vi "hydraharp_initialize_correlation.vi"(8 "error in (no error)":errorcluster, 11 "hydraharp in":refnum<class "hydraharp.lvclass">) -> (0 "error out":errorcluster, 3 "hydraharp out":refnum<class "hydraharp.lvclass">)   [LabVIEW 2015, in "hydraharp.lvclass"]
uses:
  hydraharp.lvclass
  hydraharp.lvclass/hydraharp.ctl
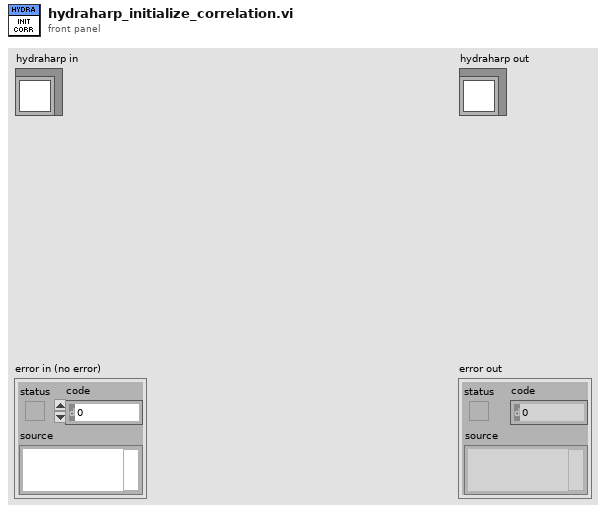
[diagram p1: front panel]
types:
  T1 = cluster{"log_bin_edges":dbl[], "ch1_photons":dbl[], "ch2_photons":dbl[], "elements_in_record_buffers":i32[], "number_of_new_photons":i32[]}
  T2 = typedef "hydraharp_correlation_lag_settings.ctl" = cluster{"time_start":T3, "time_end":T3, "coarseness":i64}
  T3 = typedef "hydraharp_time_decades.ctl" = i64
  T4 = typedef "hydraharp_action_on_records.ctl" = enum16{"stream_to_file", "correlate", "stream to file and correlate"}
  T5 = typedef "hpanel_acq_modes.ctl" = u16
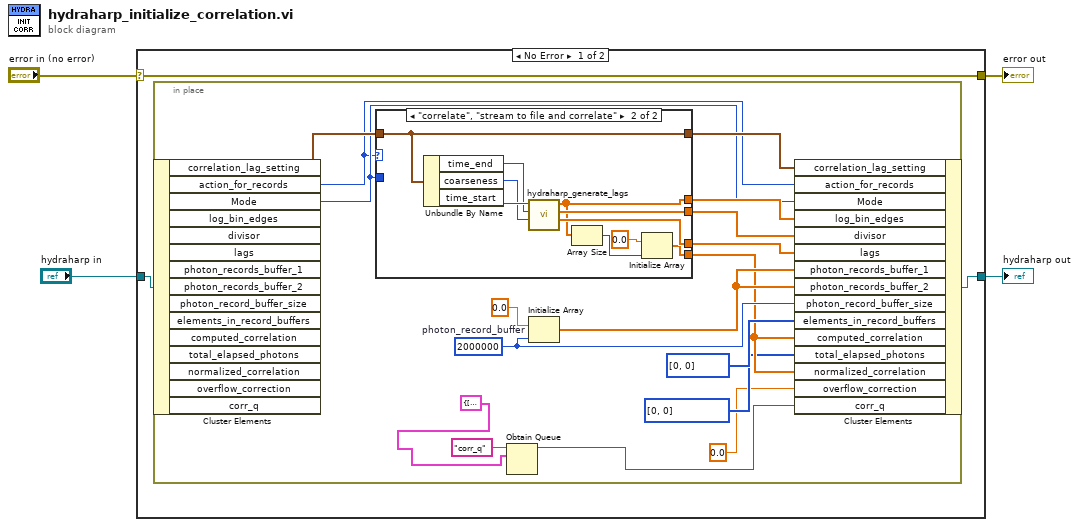
[diagram p0: block diagram]
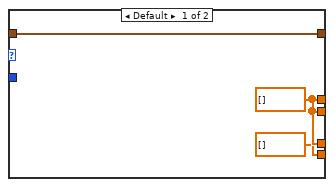
[diagram p2: hidden frame]
diagram:
  n1 = case shown="No Error" "error in (no error)" {
    selector: "error in (no error)" -> [w7 w39]
    tunnel: [w7 w39] -> w3
    tunnel: [w5 w38] -> w1
    tunnel: "hydraharp in" -> [w6 w38]
    frame No Error {
      n2 = in-place {
        w15 = 2000000 ("dimension size")
        n3 = in-place-cluster #1(w6) -> ("correlation_lag_setting"=w24:T2, "action_for_records"=w18:T4, "Mode"=w19:T5)  [unwired: 12 out]
        n4 = case shown="\"correlate\", \"stream to file and correlate\"" w18 {
          tunnel: w19 -> [_ _]
          tunnel: w24 -> [w27 w34]
          tunnel: [w27 w34] -> w23
          tunnel: [w26 w33] -> w22
          tunnel: [w26 w30] -> w21
          tunnel: [w26 w32] -> w20
          tunnel: [dbl[] [] w28] -> w13
          frame Default {
            w26 = dbl[] [] ("lags")
          }
          frame "correlate", "stream to file and correlate" {
            n5 = Unbundle By Name(w34) -> ("time_end"=w35:T3, "coarseness"=w36:i64, "time_start"=w37:T3)
            n6 = call "hydraharp_generate_lags.vi"("coarseness"=w36, "time_end"=w35, "time_start"=w37) -> ("lags"=w32:dbl[], "divisor"=w33:dbl[], "log_bin_edges"=w30:dbl[])  [unwired: 6 in]
            n7 = Array Size(array=w30) -> (size(s)=w29:i32)
            n8 = Initialize Array(0.0 ("element"), w29) -> (w28:dbl[])
          }
        }
        n9 = Obtain Queue(name (unnamed)="corr_q", element data type=T1 {"log_bin_edges"=[], "ch1_photons"=[], "ch2_photons"=[], "elements_in_record_buffers"=[], "number_of_new_photons"=[]} ("output cluster")) -> (queue out=w8:refnum<queue>)  [unwired: 3 in, 2 out]
        n10 = Initialize Array "photon_record_buffer"(0.0 ("element"), w15) -> (w16:dbl[])
        n11 = in-place-cluster #1("correlation_lag_setting"=w23, "action_for_records"=w18, "Mode"=w19, "log_bin_edges"=w21, "divisor"=w22, "lags"=w20, "photon_records_buffer_1"=w16, "photon_records_buffer_2"=w16, "photon_record_buffer_size"=w15, "elements_in_record_buffers"=i32[] [0, 0], "computed_correlation"=w13, "total_elapsed_photons"=i32[] [0, 0], "normalized_correlation"=w13, "overflow_correction"=0.0, "corr_q"=w8) -> (w5:refnum<class "hydraharp.lvclass">)
      }
    }
    frame Error {
    }
  }
  "error out" <- w3
  "hydraharp out" <- w1
